vi "Create VI By Template.vi"(7 "Modify Icon?":bool=TRUE, 8 "error in":errorcluster, 10 "Template VI Path":path=path "C:/Users/OneEd/OneDrive/Desktop/MicroPort Job/CTDB/src/db_script/DB Select Template.vi", 11 "Save as":path=path "C:/Users/OneEd/OneDrive/Desktop/MicroPort Job/CTDB/src/db_script/DB Select Template.vi") -> (0 "error out":errorcluster, 3 "Save as out":path=path "C:/Users/OneEd/OneDrive/Desktop/MicroPort Job/CTDB/src/db_script/DB Select Template.vi")   [LabVIEW 2021, in "EDT VI Script.lvlib"]
uses:
  EDT VI Script.lvlib
  <vilib>/LabVIEW Icon API/Set Text Icon/Text-Based VI Icon.lvlib
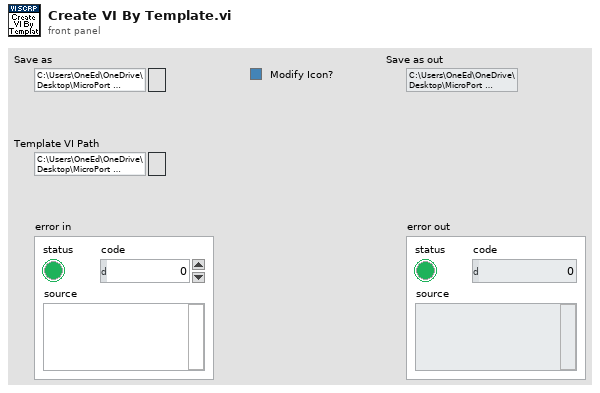
[diagram p1: front panel]
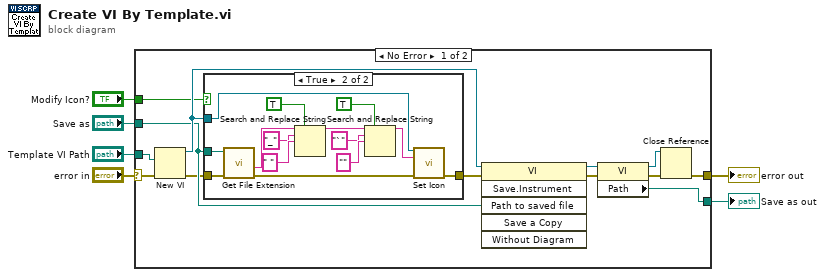
[diagram p0: block diagram]
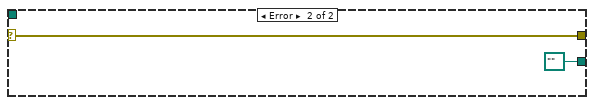
[diagram p3: hidden frame]
diagram:
  n1 = case shown="No Error" "error in" {
    selector: "error in" -> [w18 w36]
    tunnel: [w13 w36] -> w5
    tunnel: "Template VI Path" -> [w19 _]
    tunnel: [w16 path "" ("Path")] -> w3
    tunnel: "Save as" -> [w9 _]
    tunnel: "Modify Icon?" -> [w7 _]
    frame No Error {
      n2 = New VI(8:w18, 10:w19) -> (0:w8:errorcluster, 3:w10:refnum<vi>)  [unwired: 5 in]
      n3 = case shown="True" w7 {
        tunnel: [w20 w34] -> w12
        tunnel: w10 -> [_ w32]
        tunnel: w9 -> [_ w31]
        tunnel: w8 -> [w20 w30]
        frame False {
        }
        frame True {
          n4 = call <vilib>:"Get File Extension.vi"("error in (no error)"=w30, "file"=w31) -> ("error out"=w33:errorcluster, "filename without extension"=w21:string)  [unwired: 5 in, 3 out]
          n5 = Search and Replace String(replace all?=TRUE ("replace all? (F)"), input string=w21, search string="_", replace string=" " ("replace string (\"\")")) -> (result string=w26:string)  [unwired: 4 in, 3 out]
          n6 = Search and Replace String(replace all?=TRUE ("replace all? (F)"), input string=w26, search string="`", replace string="" ("replace string (\"\")")) -> (result string=w22:string)  [unwired: 4 in, 3 out]
          n7 = call <vilib>:"Set Icon.vi"("VI"=w32, "user-supplied text (\"\" - use VI file name)"=w22, "error in"=w33) -> ("error out"=w34:errorcluster)  [unwired: 11 in, 1 out]
        }
      }
      n8 = invoke class="VI" method="Save.Instrument"(reference=w10, error in=w12, "Path to saved file"=w9) -> (reference out=w17:refnum<vi>, error out=w11:errorcluster)  [unwired: 3 in, 4 out]
      n9 = property class="VI"(reference=w17, error in=w11) -> (reference out=w14:refnum<vi>, error out=w15:errorcluster, "Path"=w16:path)
      n10 = Close Reference(reference=w14, error in (no error)=w15) -> (error out=w13:errorcluster)
    }
    frame Error {
    }
  }
  "error out" <- w5
  "Save as out" <- w3
